vi "Connect Channel.vi"(6 "Custom Connection Data":variant, 8 "error in (no error)":errorcluster, 9 "Publisher Name":string, 10 "Subscriber Name":string, 11 "CIFChannelMng in":refnum<class "CIFChannelMng.lvclass">) -> (0 "error out":errorcluster, 3 "CIFChannelMng out":refnum<class "CIFChannelMng.lvclass">)   [LabVIEW 2021, in "CIFChannelMng.lvclass"]
uses:
  CIFChannelMng.lvclass
  CIFChannelMng.lvclass/CIFChannelMng.ctl
  CIFClocks/Typedef/Errors.ctl
  <vilib>/Utility/miscctls.llb/LVMapReplaceAction.ctl
  CIFCore/Common/Utilities/Append Error Location.vi
  CIFChannels/CIFChannels.lvclass
  CIFCore/Common/CIFCoreCommon.lvlib
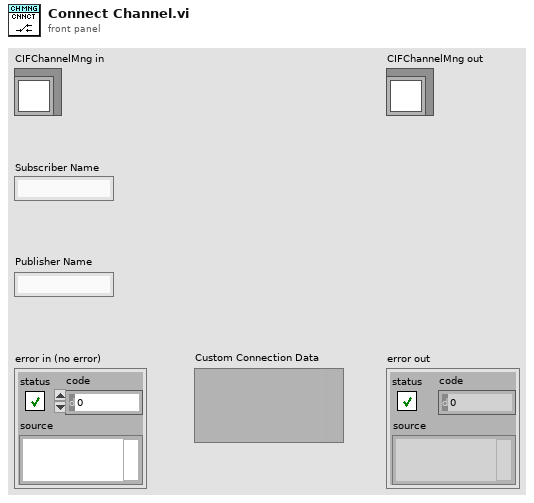
[diagram p1: front panel]
types:
  T1 = typedef "CIFCoreCommon.lvlib/Errors.ctl" = enum16{"Invalid Clock ID", "Long Sleep", "gRPC Server Not Found", "Config Parse", "Timestamp Wrap", "Delayed Execution", "Duplicate Channel", "Missing Channel", "Incorrect Type", "Unregistered Enum"}
  T2 = typedef "LVMapReplaceAction.ctl" = enum32{"Modify Entry only if found", "Add or Modify Entry", "Delete Entry"}
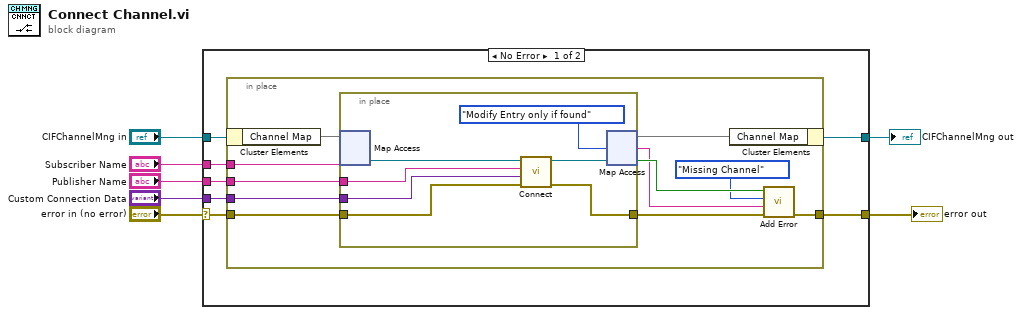
[diagram p0: block diagram]
diagram:
  n1 = case shown="No Error" "error in (no error)" {
    selector: "error in (no error)" -> [w9 w34]
    tunnel: [w8 w34] -> w6
    tunnel: [w13 w33] -> w4
    tunnel: "CIFChannelMng in" -> [w14 w33]
    tunnel: "Subscriber Name" -> [w12 _]
    tunnel: "Publisher Name" -> [w11 _]
    tunnel: "Custom Connection Data" -> [w10 _]
    frame No Error {
      n2 = in-place {
        in-place-border: w12 -> [w17]
        in-place-border: w11 -> [w23]
        in-place-border: w10 -> [w22]
        in-place-border: w9 -> [w21]
        in-place-border: [w18] -> w8
        n3 = in-place-cluster #1(w14) -> ("Channel Map"=w25:map{string, refnum<class "CIFChannels.lvclass">})
        n4 = in-place {
          in-place-border: w23 -> [w29]
          in-place-border: w22 -> [w28]
          in-place-border: w21 -> [w27]
          in-place-border: [w26] -> w19
          n5 = in-place-map #2(w25, w17) -> (w32:refnum<class "CIFChannels.lvclass">)  [unwired: 1 in, 1 out]
          n6 = call-dynamic "Connect.vi"("error in (no error)"=w27, "Custom Connection Data"=w28, "Connection Name"=w29, "CIFChannels in"=w32) -> ("error out"=w26:errorcluster, "CIFChannels out"=w31:refnum<class "CIFChannels.lvclass">)  [unwired: 6 in]
          n7 = in-place-map #2(w31, LVMapReplaceAction."Modify Entry only if found" ("action")) -> (w24:map{string, refnum<class "CIFChannels.lvclass">}, w16:string, w20:bool)
        }
        n8 = in-place-cluster #1("Channel Map"=w24) -> (w13:refnum<class "CIFChannelMng.lvclass">)
        n9 = call "Add Error.vi"("error in (no error)"=w19, "String to Append"=w16, "Error"=Errors."Missing Channel", "Insert Error"=w20) -> ("error out"=w18:errorcluster)  [unwired: 7 in]
      }
    }
    frame Error {
    }
  }
  "error out" <- w6
  "CIFChannelMng out" <- w4
